vi "simula qh.vi"(9 "%valvola":dbl, 10 "Hnom":dbl, 11 "Qnom":dbl) -> (0 "ETA simul %":dbl, 1 "P2simul [kW]":dbl, 2 "Hsimul":dbl, 3 "Qsimul[m3/h]":dbl format="%0.2f")   [LabVIEW 2016]
uses:
  <vilib>/gmath/NI_Gmath.lvlib
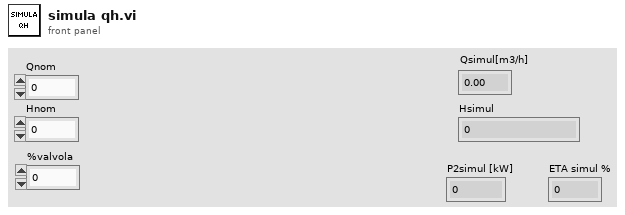
[diagram p1: front panel]
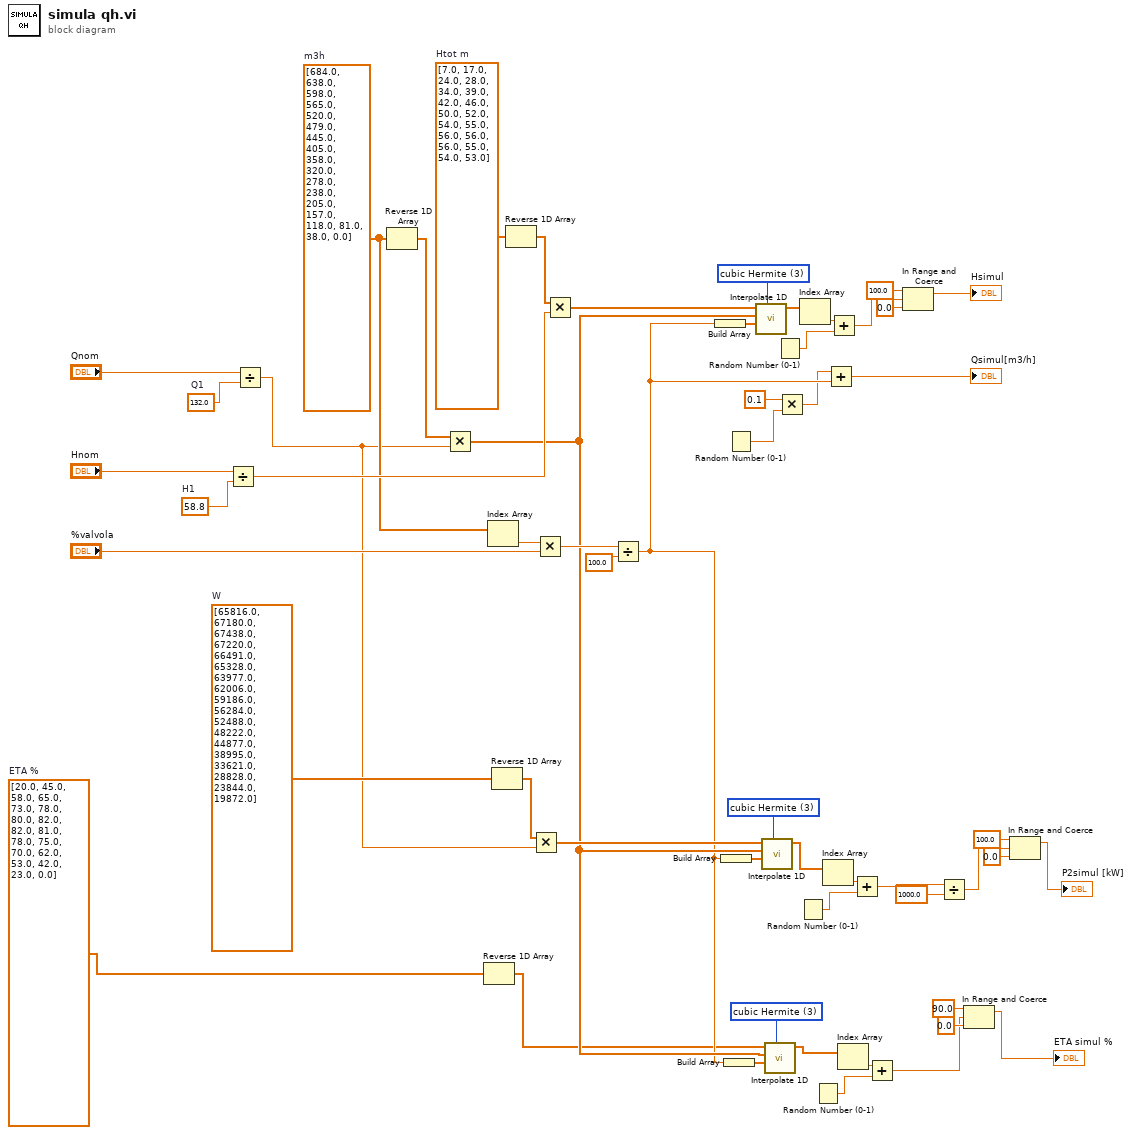
[diagram p0: block diagram]
diagram:
  w24 = 3 items=["nearest", "linear", "spline", "cubic Hermite", "Lagrange"] ("method")
  w25 = dbl[] [20.0, 45.0, 58.0, 65.0, 73.0, 78.0, 80.0, 82.0, 82.0, 81.0, 78.0, 75.0, 70.0, 62.0, 53.0, 42.0, 23.0, 0.0]  # ETA %
  w29 = 3 items=["nearest", "linear", "spline", "cubic Hermite", "Lagrange"] ("method")
  w33 = dbl[] [65816.0, 67180.0, 67438.0, 67220.0, 66491.0, 65328.0, 63977.0, 62006.0, 59186.0, 56284.0, 52488.0, 48222.0, 44877.0, 38995.0, 33621.0, 28828.0, 23844.0, 19872.0]  # W
  w39 = 3 items=["nearest", "linear", "spline", "cubic Hermite", "Lagrange"] ("method")
  w51 = dbl[] [7.0, 17.0, 24.0, 28.0, 34.0, 39.0, 42.0, 46.0, 50.0, 52.0, 54.0, 55.0, 56.0, 56.0, 56.0, 55.0, 54.0, 53.0]  # Htot m
  w44 = dbl[] [684.0, 638.0, 598.0, 565.0, 520.0, 479.0, 445.0, 405.0, 358.0, 320.0, 278.0, 238.0, 205.0, 157.0, 118.0, 81.0, 38.0, 0.0]  # m3h
  w54 = 58.8  # H1
  w55 = 132.0  # Q1
  n1 = Divide(x="Hnom", y=w54) -> (x/y=w52:dbl)
  n2 = Divide(x="Qnom", y=w55) -> (x/y=w32:dbl)
  n3 = Reverse 1D Array(array=w44) -> (reversed array=w46:dbl[])
  n4 = Multiply(x=w46, y=w32) -> (x*y=w22:dbl[])
  n5 = Reverse 1D Array(array=w25) -> (reversed array=w17:dbl[])
  n6 = Index Array(array=w44) -> (element=w38:dbl)  [unwired: 1 in]
  n7 = Reverse 1D Array(array=w33) -> (reversed array=w34:dbl[])
  n8 = Reverse 1D Array(array=w51) -> (reversed array=w45:dbl[])
  n9 = Multiply(x=w34, y=w32) -> (x*y=w30:dbl[])
  n10 = Multiply(x=w38, y="%valvola") -> (x*y=w48:dbl)
  n11 = Multiply(x=w45, y=w52) -> (x*y=w43:dbl[])
  n12 = Divide(x=w48, y=100.0) -> (x/y=w21:dbl)
  n13 = Build Array(w21) -> (w41:dbl[])
  n14 = Build Array(w21) -> (w31:dbl[])
  n15 = Build Array(w21) -> (w23:dbl[])
  n16 = Random Number (0-1)() -> (number: 0 to 1=w35:dbl)
  n17 = call <vilib>:"Interpolate 1D.vi"("method"=w39, "xi"=w41, "X"=w22, "Y"=w43) -> ("yi"=w40:dbl[])  [unwired: 5 in, 2 out]
  n18 = call <vilib>:"Interpolate 1D.vi"("method"=w29, "xi"=w31, "X"=w22, "Y"=w30) -> ("yi"=w26:dbl[])  [unwired: 5 in, 2 out]
  n19 = call <vilib>:"Interpolate 1D.vi"("method"=w24, "xi"=w23, "X"=w22, "Y"=w17) -> ("yi"=w18:dbl[])  [unwired: 5 in, 2 out]
  n20 = Random Number (0-1)() -> (number: 0 to 1=w36:dbl)
  n21 = Multiply(x=0.1, y=w35) -> (x*y=w14:dbl)
  n22 = Random Number (0-1)() -> (number: 0 to 1=w28:dbl)
  n23 = Index Array(array=w40) -> (element=w42:dbl)  [unwired: 1 in]
  n24 = Random Number (0-1)() -> (number: 0 to 1=w19:dbl)
  n25 = Index Array(array=w26) -> (element=w27:dbl)  [unwired: 1 in]
  n26 = Add(x=w14, y=w21) -> (x+y=→"Qsimul[m3/h]":dbl)
  n27 = Add(x=w42, y=w36) -> (x+y=w12:dbl)
  n28 = Index Array(array=w18) -> (element=w20:dbl)  [unwired: 1 in]
  n29 = Add(x=w27, y=w28) -> (x+y=w16:dbl)
  n30 = Add(x=w20, y=w19) -> (x+y=w2:dbl)
  n31 = In Range and Coerce(upper limit=100.0, x=w12, lower limit=0.0) -> (coerced(x)=→"Hsimul":dbl)  [unwired: 1 out]
  n32 = Divide(x=w16, y=1000.0) -> (x/y=w6:dbl)
  n33 = In Range and Coerce(upper limit=90.0, x=w2, lower limit=0.0) -> (coerced(x)=→"ETA simul %":dbl)  [unwired: 1 out]
  n34 = In Range and Coerce(upper limit=100.0, x=w6, lower limit=0.0) -> (coerced(x)=→"P2simul [kW]":dbl)  [unwired: 1 out]
